vi "SSL Vision Log Player.vi"() -> ()   [LabVIEW 2018]
uses:
  SSL Referee Game Status.ctl
  GUI/IA Robot Line Display.ctl
  Intel/Functions Enum.ctl
  Filters/Estimadores.ctl
  Control/SSL Data Control.ctl
  Control/SSL UDP Address.ctl
  Control/File Player.ctl
  Intel/Command Enum.ctl
  Test/TestModule.ctl
  Util/Select None or Robot.ctl
  DrawTargets.ctl
  Select Personalitys.ctl
  Util/Select Auto None or Robot.ctl
  Intel/AI Parameters.ctl
  grSim/grSim RobotReplacement.ctl
  grSim/grSim_BallReplacement.ctl
  SSL Detection Frame.ctl
  SSL Detection Robot.ctl
  <vilib>/Analysis/Matrix/Datatypes/RealMatrix.ctl
  SSL Detection Ball.ctl
  SSL/SSL Field State.ctl
  <extravilib>/ChannelInstances/Lossy Stream-a[.](u8)/Read With Abort.vi
  <extravilib>/ChannelInstances/Lossy Stream-t'SSL Referee Game Status.ctl'/Write With Abort.vi
  <extravilib>/ChannelInstances/Lossy Stream-bool/Read With Abort.vi
  <extravilib>/ChannelInstances/Lossy Stream-bool/Write With Abort.vi
  <extravilib>/ChannelInstances/Lossy Stream-t'AI Input.ctl'/Write With Abort.vi
  <extravilib>/ChannelInstances/Lossy Stream-c(a[.](t'grSim RobotReplacement.ctl'),t'grSim_BallReplacement.ctl')/Read With Abort.vi
  <extravilib>/ChannelInstances/Lossy Stream-t'AI Input.ctl'/Read With Abort.vi
  <extravilib>/ChannelInstances/Lossy Stream-a[.](bool)/Write With Abort.vi
  <extravilib>/ChannelInstances/Lossy Stream-a[.](i32)/Read With Abort.vi
  <extravilib>/ChannelInstances/Lossy Stream-c(a[.](t'grSim RobotReplacement.ctl'),t'grSim_BallReplacement.ctl')/Write With Abort.vi
  <extravilib>/ChannelInstances/Lossy Stream-a[.](bool)/Read With Abort.vi
  <extravilib>/ChannelInstances/Lossy Stream-a[.](u16)/Read With Abort.vi
  <extravilib>/ChannelInstances/Lossy Stream-a[.](i32)/Write With Abort.vi
  <extravilib>/ChannelInstances/Lossy Stream-t'SSL Field State.ctl'/Read With Abort.vi
  <extravilib>/ChannelInstances/Lossy Stream-t'SSL Referee Game Status.ctl'/Read With Abort.vi
  <extravilib>/ChannelInstances/Lossy Stream-a[.](t'SSL Detection Frame.ctl')/Read With Abort.vi
  <extravilib>/ChannelInstances/Lossy Stream-c(u32,u32,u32,u32,u32,u32,u32,u32,u32,u32,u32,u32,u32,u32)/Read With Abort.vi
  <extravilib>/ChannelInstances/Lossy Stream-t'SSL Field State.ctl'/Write With Abort.vi
  <extravilib>/ChannelInstances/Lossy Stream-a[.](u16)/Write With Abort.vi
  <extravilib>/ChannelInstances/Lossy Stream-a[.](t'SSL Detection Frame.ctl')/Write With Abort.vi
  <extravilib>/ChannelInstances/Lossy Stream-c(u32,u32,u32,u32,u32,u32,u32,u32,u32,u32,u32,u32,u32,u32)/Write With Abort.vi
  <extravilib>/ChannelInstances/Lossy Stream-a[.](u8)/EndpointRead.vi
  <extravilib>/ChannelInstances/Lossy Stream-t'SSL Referee Game Status.ctl'/Endpoint.vi
  <extravilib>/ChannelInstances/Lossy Stream-bool/EndpointRead.vi
  <extravilib>/ChannelInstances/Lossy Stream-bool/Endpoint.vi
  <extravilib>/ChannelInstances/Lossy Stream-t'AI Input.ctl'/Endpoint.vi
  <extravilib>/ChannelInstances/Lossy Stream-c(a[.](t'grSim RobotReplacement.ctl'),t'grSim_BallReplacement.ctl')/EndpointRead.vi
  <extravilib>/ChannelInstances/Lossy Stream-t'AI Input.ctl'/EndpointRead.vi
  <extravilib>/ChannelInstances/Lossy Stream-a[.](bool)/Endpoint.vi
  <extravilib>/ChannelInstances/Lossy Stream-a[.](i32)/EndpointRead.vi
  <extravilib>/ChannelInstances/Lossy Stream-c(a[.](t'grSim RobotReplacement.ctl'),t'grSim_BallReplacement.ctl')/Endpoint.vi
  <extravilib>/ChannelInstances/Lossy Stream-a[.](bool)/EndpointRead.vi
  <extravilib>/ChannelInstances/Lossy Stream-a[.](u16)/EndpointRead.vi
  <extravilib>/ChannelInstances/Lossy Stream-a[.](i32)/Endpoint.vi
  <extravilib>/ChannelInstances/Lossy Stream-t'SSL Field State.ctl'/EndpointRead.vi
  <extravilib>/ChannelInstances/Lossy Stream-t'SSL Referee Game Status.ctl'/EndpointRead.vi
  <extravilib>/ChannelInstances/Lossy Stream-a[.](t'SSL Detection Frame.ctl')/EndpointRead.vi
  <extravilib>/ChannelInstances/Lossy Stream-c(u32,u32,u32,u32,u32,u32,u32,u32,u32,u32,u32,u32,u32,u32)/EndpointRead.vi
  <extravilib>/ChannelInstances/Lossy Stream-t'SSL Field State.ctl'/Endpoint.vi
  <extravilib>/ChannelInstances/Lossy Stream-a[.](u16)/Endpoint.vi
  <extravilib>/ChannelInstances/Lossy Stream-a[.](t'SSL Detection Frame.ctl')/Endpoint.vi
  <extravilib>/ChannelInstances/Lossy Stream-c(u32,u32,u32,u32,u32,u32,u32,u32,u32,u32,u32,u32,u32,u32)/Endpoint.vi
  <extravilib>/ChannelInstances/Lossy Stream-a[.](t'SSL Detection Frame.ctl')/Instantiate.vi
  <extravilib>/ChannelInstances/Lossy Stream-c(u32,u32,u32,u32,u32,u32,u32,u32,u32,u32,u32,u32,u32,u32)/Instantiate.vi
  <extravilib>/ChannelInstances/Lossy Stream-a[.](u8)/Instantiate.vi
  <extravilib>/ChannelInstances/Lossy Stream-a[.](u8)/)Channel.vi
  <resource>/ChannelSupport/_ChannelSupport/WaitIfNeeded.vi
  <extravilib>/ChannelInstances/Lossy Stream-a[.](t'SSL Detection Frame.ctl')/)Channel.vi
  <extravilib>/ChannelInstances/Lossy Stream-c(u32,u32,u32,u32,u32,u32,u32,u32,u32,u32,u32,u32,u32,u32)/)Channel.vi
  <extravilib>/ChannelInstances/Lossy Stream-a[.](i32)/Instantiate.vi
  <extravilib>/ChannelInstances/Lossy Stream-t'SSL Field State.ctl'/Instantiate.vi
  Util/PreviousState.vi
  <extravilib>/ChannelInstances/Lossy Stream-c(a[.](t'grSim RobotReplacement.ctl'),t'grSim_BallReplacement.ctl')/Instantiate.vi
  <extravilib>/ChannelInstances/Lossy Stream-bool/Instantiate.vi
  <extravilib>/ChannelInstances/Lossy Stream-a[.](bool)/Instantiate.vi
  <extravilib>/ChannelInstances/Lossy Stream-t'AI Input.ctl'/Instantiate.vi
  <extravilib>/ChannelInstances/Lossy Stream-bool/)Channel.vi
  <extravilib>/ChannelInstances/Lossy Stream-t'AI Input.ctl'/)Channel.vi
  <extravilib>/ChannelInstances/Lossy Stream-a[.](bool)/)Channel.vi
  <extravilib>/ChannelInstances/Lossy Stream-a[.](i32)/)Channel.vi
  <extravilib>/ChannelInstances/Lossy Stream-c(a[.](t'grSim RobotReplacement.ctl'),t'grSim_BallReplacement.ctl')/)Channel.vi
  <extravilib>/ChannelInstances/Lossy Stream-a[.](u16)/Instantiate.vi
  <extravilib>/ChannelInstances/Lossy Stream-t'SSL Field State.ctl'/)Channel.vi
  <extravilib>/ChannelInstances/Lossy Stream-a[.](u16)/)Channel.vi
  <extravilib>/ChannelInstances/Lossy Stream-t'SSL Referee Game Status.ctl'/Instantiate.vi
  <extravilib>/ChannelInstances/Lossy Stream-t'SSL Referee Game Status.ctl'/)Channel.vi
  <extravilib>/ChannelInstances/Lossy Stream-t'SSL Referee Game Status.ctl'.lvlib
  <extravilib>/ChannelInstances/Lossy Stream-t'AI Input.ctl'.lvlib
  <extravilib>/ChannelInstances/Lossy Stream-a[.](u8).lvlib
  <vilib>/Analysis/Matrix/NI_Matrix.lvlib
  <extravilib>/ChannelInstances/Lossy Stream-a[.](i32).lvlib
  <extravilib>/ChannelInstances/Lossy Stream-t'SSL Field State.ctl'.lvlib
  <extravilib>/ChannelInstances/Lossy Stream-bool.lvlib
  <extravilib>/ChannelInstances/Lossy Stream-a[.](u16).lvlib
  <extravilib>/ChannelInstances/Lossy Stream-c(a[.](t'grSim RobotReplacement.ctl'),t'grSim_BallReplacement.ctl').lvlib
  <extravilib>/ChannelInstances/Lossy Stream-a[.](bool).lvlib
  <extravilib>/ChannelInstances/Lossy Stream-c(u32,u32,u32,u32,u32,u32,u32,u32,u32,u32,u32,u32,u32,u32).lvlib
  <extravilib>/ChannelInstances/Lossy Stream-a[.](t'SSL Detection Frame.ctl').lvlib
panel:
  in  "Robô":i32
  in  "Liga/Desliga":bool
  out "Camera Decode FPS":dbl
  out "Filter Observation FPS":dbl
  out "2D Picture":picture
  out "Direct\nkick":bool
  out "Intel FPS":dbl
  in  "CamerasToIgnore":dbl[](array[numeric])=[-1.0, -1.0, -1.0, -1.0]
  in  "Test tab control":enum32{"Modo Teste", "GrSim Modo Teste"}(tab)
  in  "test module":T1={"Goto"="None", "ZigZag 0"=["None", "None", "None", "None", "None", "None", "None", "None", "None"], "Kicker"="None", "Vel_kick"=100.0, "Kick"=FALSE, "Modo Teste?"=FALSE, "GoTo point"=[], "zigzag points"=[{"x"=300.0, "y"=2000.0}, {"x"=300.0, "y"=-2000.0}], " id vel"=1, "Dribble"=FALSE, "Gravando"=FALSE, "output xy"=4.0, "output\nangle"=4.0, "angle\nzigzag"=32.5, "output inc"=2.0, "Accel"=6.0, "DesAccel"=1.35}
  in  "Test Mode On":bool
  in  "Generate new random points":bool
  in  "Number of Points":i32=100
  in  "Replace Robots":bool=TRUE
  in  "reset":bool
  out "Completed Generation":bool
  in  "id":i32=5
  out "kick num":i32
  in  "Test Attacker":bool
  in  "Modulo Velocidade":dbl=2000.0 format="%#_13g"
  in  "Test Passe":bool
  in  "Debug":bool
  in  "GoTo Navigation":bool
  in  "Pinned":T3={"Attc"="Auto", "Strk"="Auto", "Def"=["Auto", "Auto", "Auto"]}
  in  "Draw Targets?":T5={"Attacker"=TRUE, "Striker"=TRUE, "Goalie"=TRUE, "Defender"=TRUE, "kick"=TRUE, "Est Ball"=TRUE, "Est Robot"=FALSE, "Path S"=FALSE, "Path C"=FALSE, "Dngr.Enemy"=TRUE}
  in  "SSL Data":T6={"Modo"=TRUE, "SSL UDP RX"={"Port:"=10006, "Server IP:"="224.5.23.2", "Local IP:"="10.4.0.248", "RX"=TRUE}, "RefBox UDP RX"={"Port:"=10003, "Server IP:"="224.5.23.1", "Local IP:"="10.4.0.248", "RX"=TRUE}, "Reprodução de Arquivo"={"file path (use dialog)"=path "E:/Media/2016-07-01_cmdragons_immortals.log", "size (in bytes)"=0, "offset (in bytes)"=0, "Slide"=0.0, "Play"=FALSE, "Time Stamp"=timestamp(0 s since 1904-01-01), "Playing"=FALSE}} {"Reprodução de Arquivo"."Time Stamp" format="%<%.3X %x>T"; "Reprodução de Arquivo"."Slide" min=0 max=1 scale=0.0..1.0; "Reprodução de Arquivo"."offset (in bytes)" format="%.3p"; "Reprodução de Arquivo"."size (in bytes)" format="%.3p"}
  out "error out 5":errorcluster
  out "error out 3":errorcluster
  out "Pass":bool
  out "IA command":T9
  in  "ignora esquerda?":bool
  in  "ignora lado?":bool
  in  "atacando ao contrário?":bool
  in  "Defense stretch":i32=2000
  in  "Defense width":i32=1000
  in  "Estimador":T10=enum."Kalman"
  out "Role Playing \nFPS":dbl
  out "Total Delay":dbl format="%#.5g"
  in  "Goalie":string(combo)="0"
  in  "Command":string(combo)="Auto"
  in  "Time":enum16{"Azul", "Amarelo"}(ring) caption="Enum"
  in  "Lado":enum16{"Esquerdo", "Direito"}(ring) caption="Enum"
  in  "Role Decisor":enum16{"Simple Role Decisor", "No Role Decisor"}(ring)
  out "bot velocity":dbl(graph)
  out "ball":dbl(graph)
  in  "Tab Control":enum32{"RX Info", "TX info", "AI Parameters"}(tab)=enum."AI Parameters"
  out "GUI Robot Array":T11[](array[typedef])
  out "Game Status":T13={"Stage"="Normal First Half Pre", "Command"="Stop", "Time Left"=0.0, "Yellow Team"="", "Blue Team"="", "Yellow Score"=0, "Blue Score"=0, "Yellow Red Cards"=0, "Blue Red Cards"=0, "Yellow Yellow Cards"=0, "Blue Yellow Cards"=0, "Yellow Timeouts Left"=0, "Blue Timeouts Left"=0, "Yellow Timeout Remaining"=0.0, "Blue Timeout Remaining"=0.0, "Yellow Goalie Id"=0, "Blue Goalie Id"=0, "Time"=timestamp(2082758400 s since 1904-01-01)} {"Time" format="%<%.3X %x>T"; "Blue Timeout Remaining" format="%<%M:%S>t"; "Yellow Timeout Remaining" format="%<%M:%S>t"; "Time Left" format="%<%M:%S>t"}
  in  "Serial TX":bool
  in  "UDP GrSim TX":bool=TRUE
  in  "Address:":string="127.0.0.1"
  in  "Port:":u16=20011
  in  "Porta:":refnum<visa-resource-name>
  out "Comm TX FPS":dbl
  in  "UDP SOS TX":bool
  in  "SOS Address:":string="192.168.0.101"
  in  "SOS Port:":u16=10021
  in  "SOS Port: 2":u16=10025
  out "grSim replacement":cluster{"robots":T14[], "ball":T15}
  out "replace active":bool
  in  "AI Parameters":T16={"GotoKick"={"Dist do cone a frente"=0.0, "attacker farback"=1300.0, "Perto"=300.0, "min dist to kick"=140.0, "kick eps"=0.15, "Time to transition"=0.3}, "Attacker"={"CC chute"=0.7, "CC passe"=0.65, "Kick Force"=85.0, "ball-robot Kick"=300.0, "ball-robot Pass"=350.0, "drible\nAttk"=FALSE}, "Defender"={"D max"=1500.0, "Vel p/ robô av"=0.2, "Kick Force"=100.0, "D atk-def"=400.0, "D farback"=300.0, "drible\ndef"=FALSE, "drible\ngoalie"=FALSE}, "Timeout"={"Field/v in x"=6.0, "Dist Robots"=300, "Dist up in y"=300}, "Pose Striker"={"dist"=650.0, "Numeric"=-4.0, "dist 2"=650.0, "drible\nstriker"=TRUE}, "Dist Stop"=700.0, "D ball out"=200, "D central gap "=125.0, "T pass"=5.0, "Force ++"=5.0, "range kick"=60.0, "Chute alto"=TRUE, "Marcador novo"=TRUE, "drible"=FALSE, "D drible"=500.0} {"D drible" format="%#_13g"; "D central gap" format="%#_13g"; "Dist Stop" format="%#_13g"; "Pose Striker"."Numeric" format="%#_13g"; "Defender"."Kick Force" format="%#_13g"; "Defender"."Vel p/ robô av" format="%#_13g"; "Attacker"."ball-robot Kick" format="%#_13g"; "Attacker"."Kick Force" format="%#_13g"; "Attacker"."CC passe" format="%#_13g"; "Attacker"."CC chute" format="%#_13g"; "GotoKick"."min dist to kick" format="%#_13g"; "GotoKick"."Perto" format="%#_13g"; "GotoKick"."attacker farback" format="%#_13g"; "GotoKick"."Dist do cone a frente" format="%#_13g"}
  in  "D posse":dbl=220.0
  in  "Tol ang posse":dbl=0.3
  in  "D toque":dbl=130.0
  in  "Qtd Min p/ Stk":dbl=4.0
  in  "Mais perigoso/segundo\nmais perigoso":T17(ring)
  in  "Defesa nova/antiga":T18(ring)
  in  "D bola anda":dbl=2.0
  # "Ligue o Test Mode\nprimeiro"
  # "UDP"
  # "LOG"
  # "Score"
  # "Red Cards"
  # "Yellow Cards"
  # "Timeouts Left"
  # "Timeout Remaining"
  # "Goalie ID"
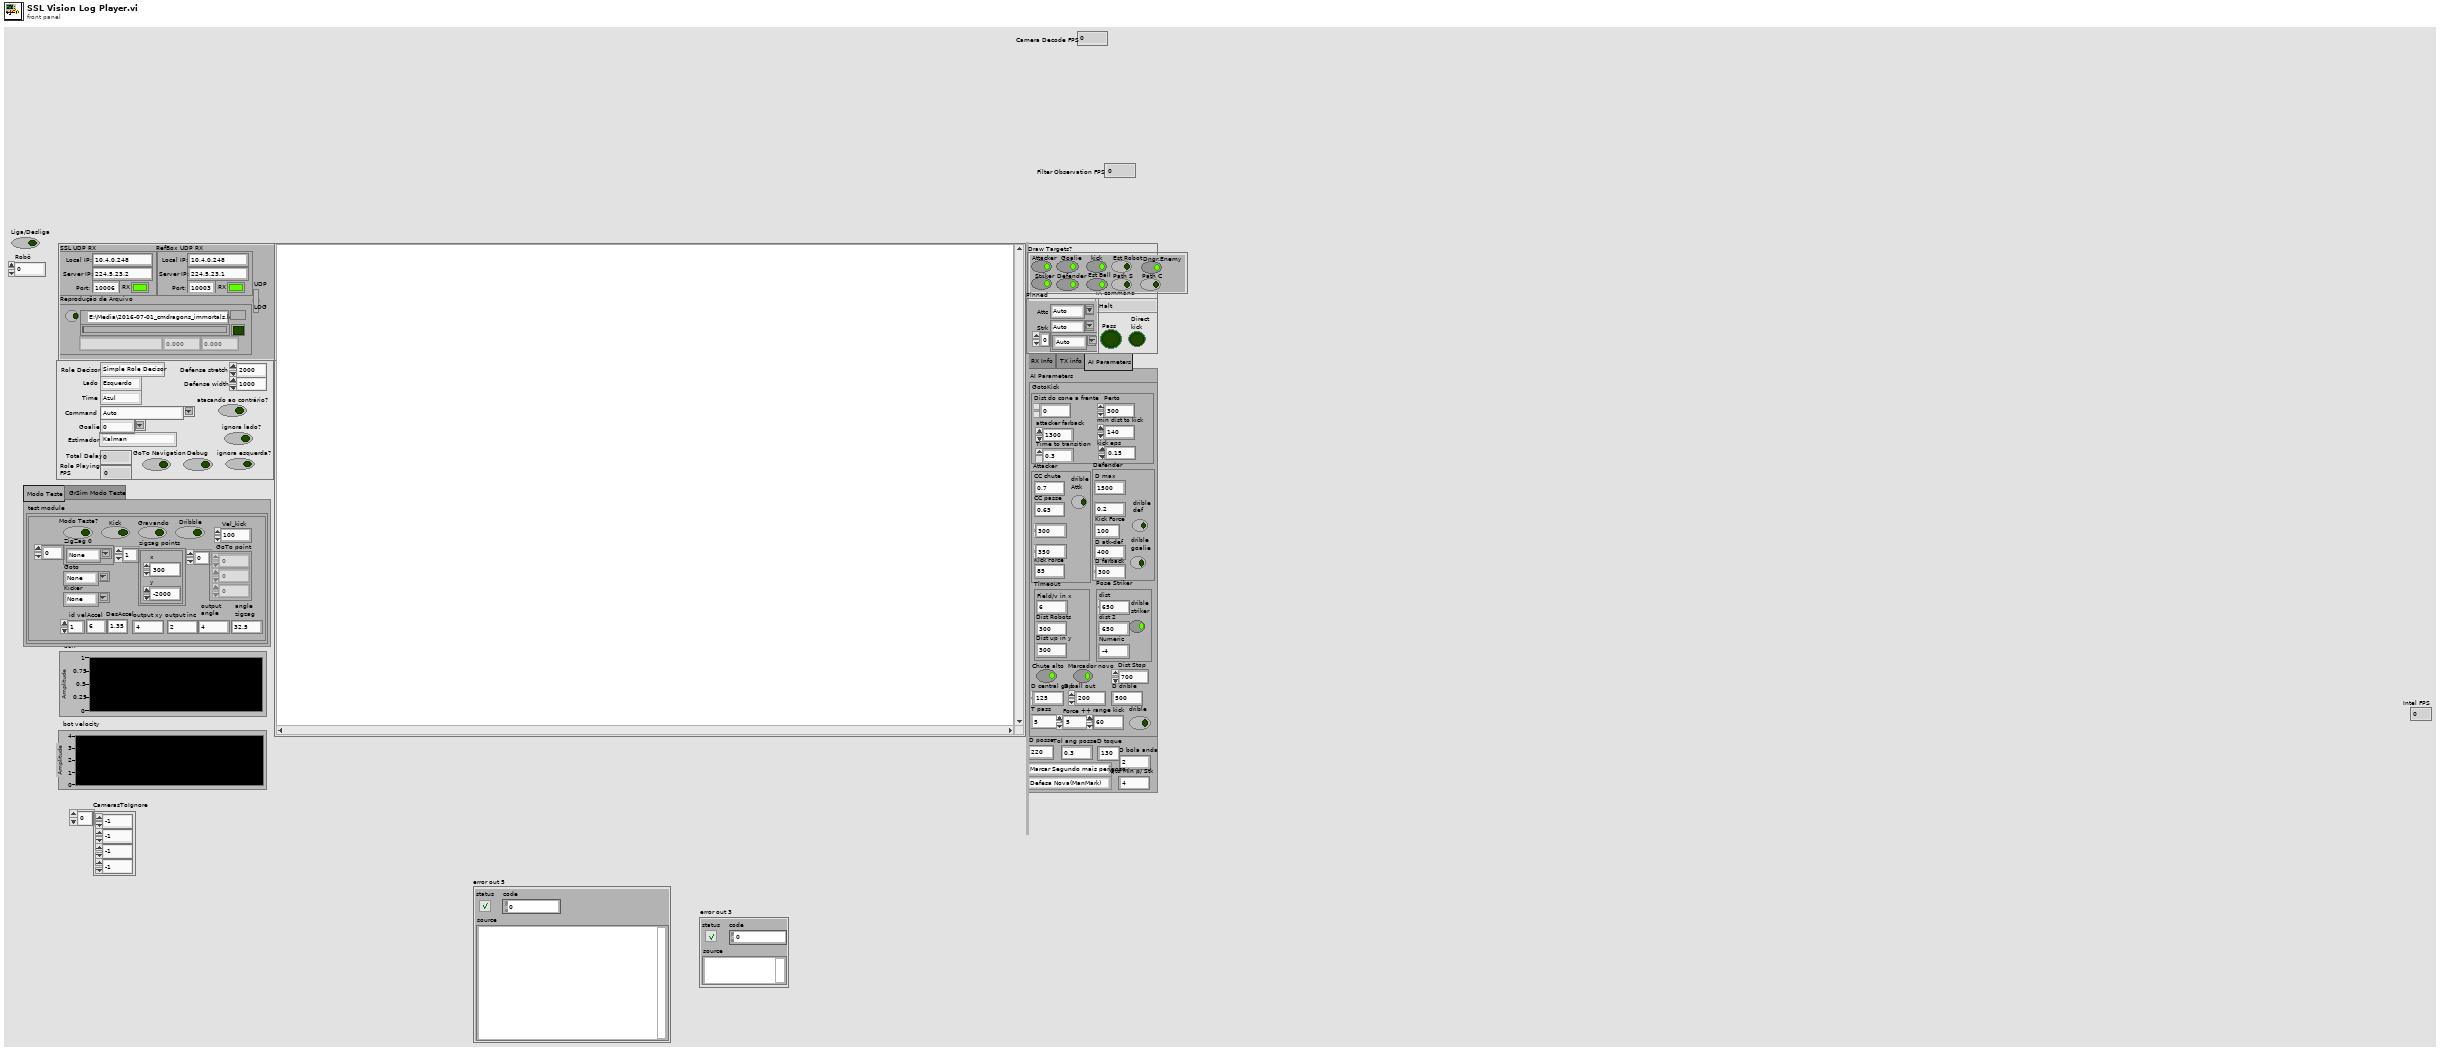
[diagram p1: front panel]
types:
  T1 = typedef "TestModule.ctl" = cluster{"Goto":T2, "ZigZag 0":T2[], "Kicker":T2, "Vel_kick":dbl, "Kick":bool, "Modo Teste?":bool, "GoTo point":dbl[], "zigzag points":cluster{"x":dbl, "y":dbl}[], " id vel":u32, "Dribble":bool, "Gravando":bool, "output xy":dbl, "output\nangle":dbl, "angle\nzigzag":dbl, "output inc":dbl, "Accel":dbl, "DesAccel":dbl}
  T2 = typedef "Select None or Robot.ctl" = string
  T3 = typedef "Select Personalitys.ctl" = cluster{"Attc":T4, "Strk":T4, "Def":T4[]}
  T4 = typedef "Select Auto None or Robot.ctl" = string
  T5 = typedef "DrawTargets.ctl" = cluster{"Attacker":bool, "Striker":bool, "Goalie":bool, "Defender":bool, "kick":bool, "Est Ball":bool, "Est Robot":bool, "Path S":bool, "Path C":bool, "Dngr.Enemy":bool}
  T6 = typedef "SSL Data Control.ctl" = cluster{"Modo":bool, "SSL UDP RX":T7, "RefBox UDP RX":T7, "Reprodução de Arquivo":T8}
  T7 = typedef "SSL UDP Address.ctl" = cluster{"Port:":u16, "Server IP:":string, "Local IP:":string, "RX":bool}
  T8 = typedef "File Player.ctl" = cluster{"file path (use dialog)":path, "size (in bytes)":i64, "offset (in bytes)":i64, "Slide":sgl, "Play":bool, "Time Stamp":timestamp, "Playing":bool}
  T9 = typedef "Command Enum.ctl" = enum16{"Halt", "Stop", "Force Start", "PKA Normal Start", "Prepare Kickoff Ally", "PKE Normal Start", "Prepare Kickoff Enemy", "Prepare Penalty Ally", "PPA Normal Start", "Prepare Penalty Enemy", "PPE Normal Start", "Direct Free Enemy", "Direct Free Ally", "Indirect Free Enemy", "Indirect Free Ally", "Timeout Enemy", "Timeout Ally", "Goal Enemy", "Goal Ally", "Ball Placement Enemy", "Ball Placement Ally", "Normal Half Time", "Extra Time Break", "Extra Half Time", "None", "Post Game"}
  T10 = typedef "Estimadores.ctl" = enum16{"Nenhum", "Simples", "Kalman"}
  T11 = typedef "IA Robot Line Display.ctl" = cluster{"ID":dbl, "function":T12, "dribble":bool}
  T12 = typedef "Functions Enum.ctl" = enum16{"Attacker", "Goalie", "Defender", "Striker", "Goto 0", "Dummy", "Kicker", "ZigZag 0", "ZigZag 1", "ZigZag 2", "ZigZag 3", "ZigZag 4", "ZigZag 5", "ZigZag 6", "ZigZag 7", "ZigZag 8", ""}
  T13 = typedef "SSL Referee Game Status.ctl" = cluster{"Stage":string, "Command":string, "Time Left":dbl, "Yellow Team":string, "Blue Team":string, "Yellow Score":u32, "Blue Score":u32, "Yellow Red Cards":u32, "Blue Red Cards":u32, "Yellow Yellow Cards":u32, "Blue Yellow Cards":u32, "Yellow Timeouts Left":u32, "Blue Timeouts Left":u32, "Yellow Timeout Remaining":dbl, "Blue Timeout Remaining":dbl, "Yellow Goalie Id":u32, "Blue Goalie Id":u32, "Time":timestamp}
  T14 = typedef "grSim RobotReplacement.ctl" = cluster{"x":dbl, "y":dbl, "dir":dbl, "yellowteam":bool, "id":u32}
  T15 = typedef "grSim_BallReplacement.ctl" = cluster{"x":dbl, "y":dbl, "vx":dbl, "vy":dbl}
  T16 = typedef "AI Parameters.ctl" = cluster{"GotoKick":cluster{"Dist do cone a frente":dbl, "attacker farback":dbl, "Perto":dbl, "min dist to kick":dbl, "kick eps":dbl, "Time to transition":dbl}, "Attacker":cluster{"CC chute":dbl, "CC passe":dbl, "Kick Force":dbl, "ball-robot Kick":dbl, "ball-robot Pass":dbl, "drible\nAttk":bool}, "Defender":cluster{"D max":dbl, "Vel p/ robô av":dbl, "Kick Force":dbl, "D atk-def":dbl, "D farback":dbl, "drible\ndef":bool, "drible\ngoalie":bool}, "Timeout":cluster{"Field/v in x":dbl, "Dist Robots":u32, "Dist up in y":u32}, "Pose Striker":cluster{"dist":dbl, "Numeric":dbl, "dist 2":dbl, "drible\nstriker":bool}, "Dist Stop":dbl, "D ball out":i32, "D central gap ":dbl, "T pass":dbl, "Force ++":dbl, "range kick":dbl, "Chute alto":bool, "Marcador novo":bool, "drible":bool, "D drible":dbl}
  T17 = enum16{"Marcar Segundo mais perigoso", "Marcar o mais perigoso"}
  T18 = enum16{"Defesa Nova(ManMark)", "Defesa Antiga(Barreira)"}
  T19 = typedef "Lossy Stream-a[.](u8).lvlib/)Channel.ctl" = refnum<queue>
  T20 = typedef "SSL Referee.ctl" = cluster{"packet_\ntimestamp":u64, "stage":u64, "stage_time_left":i32, "command ":u64, "command_\ncounter ":u32, "command_\ntimestamp":u64, "yellow team info":T21, "blue team info":T21, "Point":cluster{"x":sgl, "y":sgl}}
  T21 = typedef "SSL Referee Team Info.ctl" = cluster{"name":string, "score":u32, "red_cards":u32, "yellow_cards_time":u32[], "yellow_cards":u32, "timeout":u32, "timeout_times":u32, "goalie":u32}
  T22 = typedef "Lossy Stream-t'SSL Referee Game Status.ctl'.lvlib/)Channel.ctl" = refnum<queue>
  T23 = typedef "SSL Detection Frame.ctl" = cluster{"frame_number":u32, "t_capture":dbl, "t_sent":dbl, "camera_id":u32, "robots_yellow":T24[], "robots_blue":T24[], "balls":T26[], "Valid":bool, "Time Stamp":timestamp}
  T24 = typedef "SSL Detection Robot.ctl" = cluster{"x":sgl, "robot_id":u32, "confidence":sgl, "y":sgl, "orientation":sgl, "pixel_x":sgl, "pixel_y":sgl, "height":sgl, "Valid":bool, "Time Stamp":timestamp, "x_k|k":T25, "Pk|k":T25, "Previous Time Stamp":timestamp, "R":T25}
  T25 = typedef "NI_Matrix.lvlib/RealMatrix.ctl" = dbl[][]
  T26 = typedef "SSL Detection Ball.ctl" = cluster{"x":sgl, "area":u32, "confidence":sgl, "y":sgl, "z":sgl, "pixel_x":sgl, "pixel_y":sgl, "Valid":bool, "Time Stamp":timestamp, "x_k|k":T25, "Pk|k":T25, "Id":u32, "Previous Time Stamp":timestamp, "R":T25}
  T27 = cluster{"line_width":u32, "field_length":u32, "field_width":u32, "boundary_width":u32, "referee_width":u32, "goal_width":u32, "goal_depth":u32, "goal_wall_width":u32, "center_circle_radius":u32, "defense_radius":u32, "defense_stretch":u32, "free_kick_from_defense_dist":u32, "penalty_spot_from_field_line_dist":u32, "penalty_line_from_spot_dist":u32}
  T28 = typedef "Lossy Stream-c(u32,u32,u32,u32,u32,u32,u32,u32,u32,u32,u32,u32,u32,u32).lvlib/)Channel.ctl" = refnum<queue>
  T29 = typedef "Lossy Stream-a[.](t'SSL Detection Frame.ctl').lvlib/)Channel.ctl" = refnum<queue>
  T30 = typedef "SSL Field State.ctl" = cluster{"Detection Frame Out":T23, "Field Size Out":cluster{"line_width":u32, "field_length":u32, "field_width":u32, "boundary_width":u32, "referee_width":u32, "goal_width":u32, "goal_depth":u32, "goal_wall_width":u32, "center_circle_radius":u32, "defense_radius":u32, "defense_stretch":u32, "free_kick_from_defense_dist":u32, "penalty_spot_from_field_line_dist":u32, "penalty_line_from_spot_dist":u32}, "Received Time Stamp":timestamp}
  T31 = typedef "AI Input.ctl" = cluster{"our_robots":T32[], "enemy_robots":T32[], "balls":T36[], "geometry":T37, "IA Judge":T38, "Received Timestamp":timestamp, "Events":T39}
  T32 = typedef "AI Robot.ctl" = cluster{"id":u32, "function":T12, "x":dbl, "y":dbl, "orientation":dbl, "v_tangent":dbl, "v_normal":dbl, "v_ang":dbl, "kick_x":dbl, "kick_z":dbl, "dribble":bool, "Timestamp":timestamp, "estimatives":cluster{"est_v_tangent":dbl, "est_v_normal":dbl, "est_vx":dbl, "est_vy":dbl, "Pos Robot Est":dbl[]}, "dest_x_kick":dbl, "dest_y_kick":dbl, "Gap Coord":dbl[], "States":T33, "Path ":dbl[][], "Path  Smooth":dbl[][], "Dest":T34}
  T33 = typedef "AttackerStates.ctl" = enum16{"Pass", "GoToTangent", "BallGetting", "GoToKick", ""}
  T34 = typedef "PathDests.ctl" = T35[]
  T35 = typedef "PathDest.ctl" = cluster{"dest_x":dbl, "dest_y":dbl, "dest_orientation":dbl, "dest_vel":dbl}
  T36 = typedef "AI Ball.ctl" = cluster{"x":dbl, "y":dbl, "timestamp":timestamp, "Vel_x":dbl, "Vel_y":dbl, "Pos Bola Est":dbl[]}
  T37 = typedef "Field Size.ctl" = cluster{"line_width":u32, "field_length":u32, "field_width":u32, "boundary_width":u32, "referee_width":u32, "goal_width":u32, "goal_depth":u32, "goal_wall_width":u32, "center_circle_radius":u32, "defense_radius":u32, "defense_stretch":u32, "free_kick_from_defense_dist":u32, "penalty_spot_from_field_line_dist":u32, "penalty_line_from_spot_dist":u32}
  T38 = typedef "AI Judge.ctl" = cluster{"stage":string, "command":string, "our_goalie_id":dbl, "enemy_goalie_id":dbl, "command enum":T9, "Time":enum16{"Azul", "Amarelo"}}
  T39 = typedef "Events.ctl" = cluster{"Touch":bool, "Ball out":bool, "id touch":dbl, "Ball out of \nVision":bool, "Ball inside \nGoalie area":bool, "Robot not responding":bool, "Robots responding status":dbl[], "Enemy Ball \nPossession":bool, "Pass State":bool, "id end of pass":dbl, "Kick":bool, "Id ini Possession":dbl, "Ball Possesion":bool, "Id Possesion":dbl, "Direct Kick":bool}
  T40 = typedef "Lossy Stream-a[.](u16).lvlib/)Channel.ctl" = refnum<queue>
  T41 = typedef "Lossy Stream-t'SSL Field State.ctl'.lvlib/)Channel.ctl" = refnum<queue>
  T42 = typedef "Lossy Stream-a[.](i32).lvlib/)Channel.ctl" = refnum<queue>
  T43 = typedef "Lossy Stream-t'AI Input.ctl'.lvlib/)Channel.ctl" = refnum<queue>
  T44 = typedef "Lossy Stream-bool.lvlib/)Channel.ctl" = refnum<queue>
  T45 = typedef "Lossy Stream-a[.](bool).lvlib/)Channel.ctl" = refnum<queue>
  T46 = typedef "Lossy Stream-c(a[.](t'grSim RobotReplacement.ctl'),t'grSim_BallReplacement.ctl').lvlib/)Channel.ctl" = refnum<queue>
  T47 = typedef "grSim Robot Command.ctl" = cluster{"id":u32, "kickspeedx":sgl, "kickspeedz":sgl, "veltangent":sgl, "velnormal":sgl, "velangular":sgl, "spinner":bool, "wheelspeed":bool, "wheel1":sgl, "wheel2":sgl, "wheel3":sgl, "wheel4":sgl}
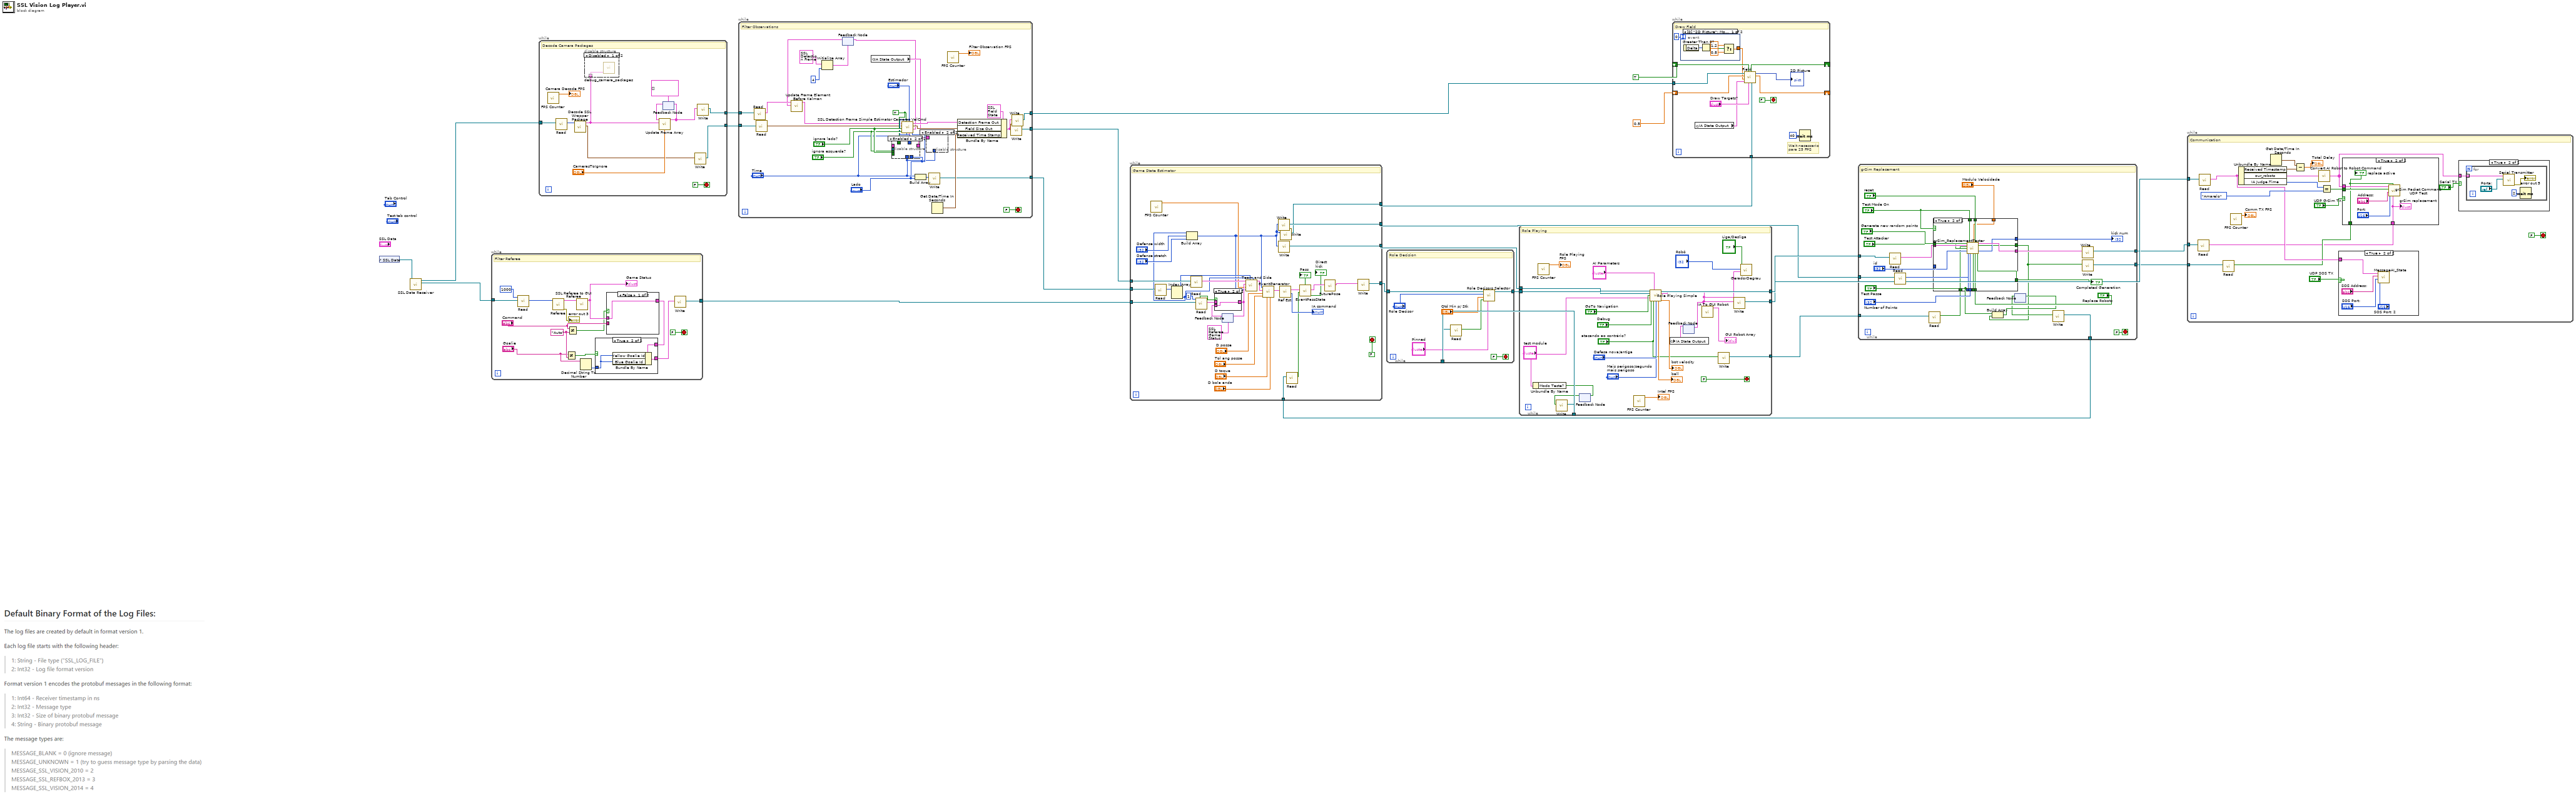
[diagram p0: block diagram]
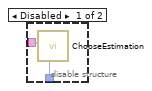
[diagram p3: hidden frame]
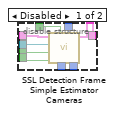
[diagram p4: hidden frame]
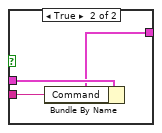
[diagram p6: hidden frame]
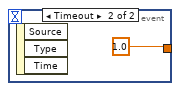
[diagram p7: hidden frame]
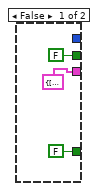
[diagram p9: hidden frame]
diagram:
  n1 = control-ref of="SSL Data"() -> (w18:refnum<vi>)
  n2 = call "SSL Data Receiver.vi"("SSL Data 2"=w18) -> ("SSL RefBox"=w19:T19, "SSL Vision"=w3:T19)  [unwired: 9 in]
  n3 = while {
    tunnel: w19 -> [w26]
    tunnel: [w36] -> w21
    stop <- FALSE stop-if-true
    w32 = "Auto" ("y")
    # "Filter Referee"
    n4 = call <extravilib>:"Read.vi"("channel"=w26, "timeout in ms (-1)"=1000) -> ("element"=w25:u8[])  [unwired: 4 in, 5 out]
    n5 = call "Referee.vi"("element"=w25) -> ("output cluster"=w37:T20, "error out"=→"error out 3":errorcluster)  [unwired: 13 in]
    n6 = Not Equal?(x="Goalie", y=w32) -> (x != y?=w31:bool)
    n7 = Not Equal?(x="Command", y=w32) -> (x != y?=w33:bool)
    n8 = call "SSL Referee to GUI Referee.vi"("SSL Game Status"=w37) -> ("GUI Game Status"=w35:T13)  [unwired: 10 in]
    "Game Status" <- w35
    n9 = Decimal String To Number(string="Goalie") -> (number=w27:i32)  [unwired: 2 in, 1 out]
    n10 = case shown="False" w33 {
      tunnel: w35 -> [w44 w47]
      tunnel: [w44 w46] -> w30
      tunnel: "Command" -> [_ w45]
      frame False {
      }
      frame True {
        n11 = Bundle By Name(cluster=w47, "Command"=w45) -> (w46:T13)
      }
    }
    n12 = case shown="True" w31 {
      tunnel: w30 -> [w40 w43]
      tunnel: [w40 w42] -> w29
      tunnel: w27 -> [_ w41]
      frame False {
      }
      frame True {
        n13 = Bundle By Name(cluster=w43, "Yellow Goalie Id"=w41, "Blue Goalie Id"=w41) -> (w42:T13)
      }
    }
    n14 = call <extravilib>:"Write.vi"("element"=w29) -> ("channel"=w36:T22)  [unwired: 8 in, 2 out]
  }
  n15 = while {
    tunnel: w3 -> [w58]
    tunnel: [w54] -> w2
    tunnel: [w53] -> w1
    stop <- FALSE stop-if-true
    # "Decode Camera Packages"
    n16 = call "FPS Counter.vi"() -> ("Numeric"=→"Camera Decode FPS":dbl)  [unwired: 11 in]
    n17 = call <extravilib>:"Read.vi"("channel"=w58) -> ("element"=w59:u8[])  [unwired: 5 in, 5 out]
    n18 = call "Decode SSL Wrapper Package.vi"("unsigned byte array"=w59) -> ("Field Size"=w55:T27, "Detection Frame"=w49:T23)  [unwired: 7 in, 2 out]
    n19 = disable-structure shown="Disabled" {
      disable-tunnel: w49 -> [w60 _]
      frame Disabled {
        n20 = call "debug_camera_packages.vi"("Detection Frame"=w60) -> ()  [unwired: 11 in]
      }
      frame Enabled {
      }
    }
    n21 = feedback #1(T23[] [] ("element")) -> (w51:T23[])
    n22 = call "Update Frame Array.vi"("CamerasToIgnore"="CamerasToIgnore", "Detection Frame In"=w49, "Array Detection Frame In"=w51) -> ("Detection Frame In out"=w48:T23[])  [unwired: 8 in]
    n23 = feedback-in #1(w48) -> ()
    n24 = call <extravilib>:"Write.vi"("element"=w55) -> ("channel"=w54:T28)  [unwired: 8 in, 2 out]
    n25 = call <extravilib>:"Write.vi"("element"=w48) -> ("channel"=w53:T29)  [unwired: 8 in, 2 out]
  }
  n26 = while {
    tunnel: [w85] -> w14
    tunnel: [w84] -> w13
    tunnel: [w73] -> w5
    tunnel: w2 -> [w71]
    tunnel: w1 -> [w69]
    stop <- FALSE stop-if-true
    w79 = TRUE ("Enable")
    # "Filter Observations"
    n27 = call <extravilib>:"Read.vi"("channel"=w69) -> ("element"=w66:T23[])  [unwired: 5 in, 5 out]
    n28 = call <extravilib>:"Read.vi"("channel"=w71) -> ("element"=w70:T27)  [unwired: 5 in, 5 out]
    n29 = Initialize Array(T23 {"frame_number"=0, "t_capture"=0.0, "t_sent"=0.0, "camera_id"=0, "robots_yellow"=[], "robots_blue"=[], "balls"=[], "Valid"=FALSE, "Time Stamp"=timestamp(0 s since 1904-01-01)} ("Detection Frame"), 4 ("dimension size")) -> (w61:T23[])
    n30 = feedback #2(w61) -> (w64:T23[])
    n31 = call "Update Frame Element Before Kalman.vi"("Old Array With Kalman"=w64, "New Array"=w66) -> ("Detection Frame In out"=w65:T23[])  [unwired: 9 in]
    n32 = global read "PreviousState.vi" "IA State Output"() -> (w68:T31)
    n33 = disable-structure shown="Enabled" {
      disable-tunnel: _ -> [w100 _]
      disable-tunnel: _ -> [w99 _]
      disable-tunnel: "ignora lado?" -> [w98 _]
      disable-tunnel: "ignora esquerda?" -> [w97 _]
      disable-tunnel: "Estimador" -> [w96 _]
      disable-tunnel: w79 -> [w95 _]
      disable-tunnel: [w94 _] -> w78
      disable-tunnel: "Lado" -> [w93 _]
      disable-tunnel: "Time" -> [w92 _]
      frame Disabled {
        n34 = call "SSL Detection Frame Simple Estimator Cameras.vi"("Lado"=w93, "Estimador"=w96, "Time"=w92, "Enable"=w95, "ignora esquerda?"=w97, "ignora lado?"=w98, "Field Size"=w99, "Detection Frame In"=w100) -> ("Detection Frame Out"=w94:T23)  [unwired: 2 in, 1 out]
      }
      frame Enabled {
      }
    }
    n35 = call "SSL Detection Frame Simple Estimator Cameras VelCmd.vi"("Lado"="Lado", "IA State Input"=w68, "Estimador"="Estimador", "Time"="Time", "Enable"=w79, "ignora esquerda?"="ignora esquerda?", "ignora lado?"="ignora lado?", "Field Size"=w70, "Detection Frame In"=w65) -> ("Frame Array"=w67:T23[], "Field Size Out"=w86:T27, "Detection Frame Out"=w75:T23)
    n36 = feedback-in #2(w67) -> ()
    n37 = Build Array("Time", "Lado") -> (w83:u16[])
    n38 = disable-structure shown="Enabled" {
      disable-tunnel: w78 -> [w91 _]
      disable-tunnel: "Time" -> [w90 _]
      frame Disabled {
        n39 = call "ChooseEstimation.vi"("Time"=w90, "Detection Frame Kalman"=w91) -> ()  [unwired: 9 in, 1 out]
      }
      frame Enabled {
      }
    }
    n40 = call <extravilib>:"Write.vi"("element"=w83) -> ("channel"=w84:T40)  [unwired: 8 in, 2 out]
    n41 = Get Date/Time In Seconds() -> (seconds since 1Jan1904=w87:timestamp)
    n42 = call "FPS Counter.vi"() -> ("Numeric"=→"Filter Observation FPS":dbl)  [unwired: 11 in]
    n43 = Bundle By Name(cluster=T30 {"Detection Frame Out"={"frame_number"=0, "t_capture"=0.0, "t_sent"=0.0, "camera_id"=0, "robots_yellow"=[], "robots_blue"=[], "balls"=[], "Valid"=FALSE, "Time Stamp"=timestamp(0 s since 1904-01-01)}, "Field Size Out"={"line_width"=0, "field_length"=0, "field_width"=0, "boundary_width"=0, "referee_width"=0, "goal_width"=0, "goal_depth"=0, "goal_wall_width"=0, "center_circle_radius"=0, "defense_radius"=0, "defense_stretch"=0, "free_kick_from_defense_dist"=0, "penalty_spot_from_field_line_dist"=0, "penalty_line_from_spot_dist"=0}, "Received Time Stamp"=timestamp(0 s since 1904-01-01)}, "Detection Frame Out"=w75, "Field Size Out"=w86, "Received Time Stamp"=w87) -> (w74:T30)
    n44 = call <extravilib>:"Write.vi"("element"=w74) -> ("channel"=w85:T41)  [unwired: 8 in, 2 out]
    n45 = call <extravilib>:"Write.vi"("element"=w74) -> ("channel"=w73:T41)  [unwired: 8 in, 2 out]
  }
  n46 = while {
    tunnel: w21 -> [w135]
    tunnel: [w129] -> w17
    tunnel: [w122] -> w15
    tunnel: w14 -> [w114]
    tunnel: w13 -> [w112]
    tunnel: w10 -> [w105]
    tunnel: [w103] -> w6
    tunnel: [w101] -> w4
    stop <- FALSE stop-if-true
    # "Game State Estimator"
    n47 = call "FPS Counter.vi"() -> ("Numeric"=w107:dbl)  [unwired: 11 in]
    n48 = call <extravilib>:"Read.vi"("channel"=w112) -> ("element"=w111:u16[])  [unwired: 5 in, 5 out]
    n49 = Index Array(array=w111) -> (element #1=w110:u16, element #2=w109:u16)  [unwired: 2 in]
    n50 = Build Array(w109, "Defense width", "Defense stretch") -> (w102:i32[])
    n51 = call <extravilib>:"Read.vi"("channel"=w114) -> ("element"=w113:T30)  [unwired: 5 in, 5 out]
    n52 = call <extravilib>:"Read.vi"("channel"=w135, "timeout in ms (-1)"=1) -> ("element"=w132:T13, "timed out?"=w133:bool)  [unwired: 4 in, 4 out]
    n53 = feedback #3(T13 {"Stage"="First Half", "Command"="Stop", "Time Left"=0.0, "Yellow Team"="", "Blue Team"="", "Yellow Score"=0, "Blue Score"=0, "Yellow Red Cards"=0, "Blue Red Cards"=0, "Yellow Yellow Cards"=0, "Blue Yellow Cards"=0, "Yellow Timeouts Left"=0, "Blue Timeouts Left"=0, "Yellow Timeout Remaining"=0.0, "Blue Timeout Remaining"=0.0, "Yellow Goalie Id"=0, "Blue Goalie Id"=0, "Time"=timestamp(0 s since 1904-01-01)} ("element")) -> (w131:T13)
    n54 = case shown="True" w133 {
      tunnel: w132 -> [w137 _]
      tunnel: [w137 w138] -> w130
      tunnel: w131 -> [_ w138]
      frame False {
      }
      frame True {
      }
    }
    n55 = feedback-in #3(w130) -> ()
    n56 = call "Team and Side.vi"("Lado"=w109, "Time"=w110, "field defense"=w102, "Comm RX FPS"=w107, "Game Status"=w130, "Field State Input"=w113) -> ("IA State"=w127:T31)  [unwired: 5 in]
    n57 = call "EventGenerator.vi"("D bola anda"="D bola anda", "Dist Para Toque"="D toque", "Tol para ang posse"="Tol ang posse", "Dist Para posse"="D posse", "IA State Input"=w127, "lado, readius, stretch"=w102) -> ("IA State Output"=w126:T31)  [unwired: 5 in]
    n58 = call <extravilib>:"Write.vi"("element"=w102) -> ("channel"=w103:T42)  [unwired: 8 in, 2 out]
    n59 = call <extravilib>:"Write.vi"("element"=w102) -> ("channel"=w122:T42)  [unwired: 8 in, 2 out]
    n60 = call "Ref Est.vi"("IA State Input"=w126) -> ("IA command"=→"IA command":T9, "IA State Output"=w121:T31)  [unwired: 9 in]
    n61 = call <extravilib>:"Write.vi"("element"=w102) -> ("channel"=w101:T42)  [unwired: 8 in, 2 out]
    n62 = call <extravilib>:"Read.vi"("channel"=w105) -> ("element"=w104:bool[])  [unwired: 5 in, 5 out]
    n63 = call "EventPassState.vi"("TestPasse"=w104, "IA State Input"=w121) -> ("Direct\nkick"=→"Direct\nkick":bool, "IA State Output"=w118:T31, "Pass State"=→"Pass":bool)  [unwired: 6 in, 1 out]
    n64 = call "FuturePose.vi"("IA State Input"=w118) -> ("output cluster"=w119:T31)  [unwired: 10 in]
    n65 = call <extravilib>:"Write.vi"("element"=w119) -> ("channel"=w129:T43)  [unwired: 8 in, 2 out]
  }
  n66 = while {
    shift-right: [w150] -> _
    shift-left: 0.5 ("New Scale") -> [w146]
    shift-right: [w149] -> _
    shift-left: TRUE ("AutoScale Out") -> [w148]
    tunnel: w4 -> [w145]
    tunnel: w5 -> [w143]
    stop <- FALSE stop-if-true
    # "Wait necessario\npara 25 FPS"
    # "Draw Field"
    n67 = event shown="[0] \"2D Picture\": Mouse Wheel" {
      selector: _ -> [_ _]
      dyn-events: _ -> [_ _]
      timeout: 0 -> [_ _]
      tunnel: [w152 1.0] -> w139
      event "2D Picture": Mouse Wheel {
        n68 = event-data() -> ("Delta"=w156:i32)  [unwired: 1 in]
        n69 = Greater Than 0?(x=w156) -> (x > 0?=w155:bool)
        n70 = Select(t=1.2, s=w155, f=0.8) -> (s? t:f=w152:dbl)
      }
      event Timeout {
        n71 = event-data() -> ()  [unwired: 1 in, 3 out]
      }
    }
    n72 = global read "PreviousState.vi" "IA State Output"() -> (w142:T31)
    n73 = call "Field.vi"("channel 2"=w145, "Draw Targets?"="Draw Targets?", "AutoScale"=w148, "IA State Output"=w142, "Zoom"=w139, "Scale mm/pixel"=w146, "channel"=w143) -> ("Scale Out"=w150:dbl, "2D Picture"=→"2D Picture":picture, "AutoScale Out"=w149:bool)  [unwired: 2 in]
    n74 = Wait (ms)(milliseconds to wait=u32 40) -> ()  [unwired: 1 out]
  }
  n75 = while {
    tunnel: w17 -> [w163]
    tunnel: [w162] -> w16
    tunnel: w12 -> [w160]
    stop <- FALSE stop-if-true
    # "Role Decision"
    n76 = call <extravilib>:"Read.vi"("channel"=w160) -> ("element"=w159:bool)  [unwired: 5 in, 5 out]
    n77 = call "Role Decisors Selector.vi"("Pinned"="Pinned", "Modo Teste ?"=w159, "Qtd Min p/ Stk"="Qtd Min p/ Stk", "Role Decisor"="Role Decisor", "channel"=w163) -> ("channel"=w162:T43)  [unwired: 5 in, 1 out]
  }
  n78 = while {
    tunnel: w16 -> [w189]
    tunnel: [w188] -> w20
    tunnel: w15 -> [w185]
    tunnel: [w176] -> w9
    tunnel: [w172] -> w12
    tunnel: [w170] -> w11
    stop <- FALSE stop-if-true
    # "Role Playing"
    n79 = Unbundle By Name("test module") -> ("Modo Teste?"=w174:bool)
    n80 = call "FPS Counter.vi"() -> ("Numeric"=→"Role Playing \nFPS":dbl)  [unwired: 11 in]
    n81 = feedback #4() -> (w173:bool)  [unwired: 1 in]
    n82 = call <extravilib>:"Write.vi"("element"=w173) -> ("channel"=w172:T44)  [unwired: 8 in, 2 out]
    n83 = feedback-in #4(w174) -> ()
    n84 = call "FPS Counter.vi"() -> ("Numeric"=→"Intel FPS":dbl)  [unwired: 11 in]
    n85 = call "Role Playing Simple.vi"(0:"channel"=w189, "AI Parameters"="AI Parameters", "Mais perigoso/segundo mais perigoso"="Mais perigoso/segundo\nmais perigoso", 5:"channel"=w185, "GoTo Navigation"="GoTo Navigation", "test module"="test module", "Debug"="Debug", "atacando ao contrário?"="atacando ao contrário?", "Defesa nova/antiga"="Defesa nova/antiga") -> ("channel"=w188:T43, "IA State Output"=w168:T31, "ball"=→"ball":dbl, "Robot"=→"bot velocity":dbl)  [unwired: 2 in, 1 out]
    n86 = feedback #5() -> (w179:T31)  [unwired: 1 in]
    n87 = global write "PreviousState.vi" "IA State Output"(w179) -> ()
    n88 = feedback-in #5(w168) -> ()
    n89 = call "IA To GUI Robot.vi"("Output IA"=w168) -> ("GUI Robot Array"=→"GUI Robot Array":T11[])  [unwired: 10 in]
    n90 = call <extravilib>:"Write.vi"("element"="atacando ao contrário?") -> ("channel"=w176:T44)  [unwired: 8 in, 2 out]
    n91 = call <extravilib>:"Write.vi"("element"=w168) -> ("channel"=w170:T43)  [unwired: 8 in, 2 out]
    n92 = call "GeradorDegrau.vi"("IA State Input"=w168, "Robô"="Robô", "Liga/Desliga"="Liga/Desliga") -> ()  [unwired: 9 in]
  }
  n93 = while {
    tunnel: [w215] -> w8
    tunnel: [w214] -> w7
    tunnel: w6 -> [w213]
    tunnel: [w198] -> w10
    tunnel: w11 -> [w195]
    tunnel: w9 -> [w193]
    stop <- FALSE stop-if-true
    # "grSim Replacement"
    n94 = call <extravilib>:"Read.vi"("channel"=w195) -> ("element"=w210:T31)  [unwired: 5 in, 5 out]
    n95 = call <extravilib>:"Read.vi"("channel"=w213) -> ("element"=w209:i32[])  [unwired: 5 in, 5 out]
    n96 = call <extravilib>:"Read.vi"("channel"=w193) -> ("element"=w194:bool)  [unwired: 5 in, 5 out]
    n97 = case shown="True" "Test Mode On" {
      tunnel: [cluster{"robots":T14[], "ball":T15} {"robots"=[], "ball"={"x"=0.0, "y"=0.0, "vx"=0.0, "vy"=0.0}} ("grSim replacement") w234] -> w211
      tunnel: w210 -> [_ w233]
      tunnel: w209 -> [_ w232]
      tunnel: "id" -> [_ w231]
      tunnel: "Generate new random points" -> [_ w230]
      tunnel: "Test Mode On" -> [_ w229]
      tunnel: "Number of Points" -> [_ w228]
      tunnel: "reset" -> [_ w227]
      tunnel: "Replace Robots" -> [_ w226]
      tunnel: [_ w225] -> w203
      tunnel: [FALSE ("Completed Generation") w224] -> w202
      tunnel: "Test Attacker" -> [_ w223]
      tunnel: "Modulo Velocidade" -> [_ w222]
      tunnel: [FALSE ("Replace active") w221] -> w191
      tunnel: "Test Passe" -> [_ w220]
      tunnel: w194 -> [_ w219]
      frame False {
      }
      frame True {
        n98 = call "grSim_ReplacementTester.vi"("Generate new random points"=w230, "IA State"=w233, "Atacando contra?"=w219, "Test Attacker"=w223, "id"=w231, "Field defense"=w232, "Test Mode On"=w229, "Number of Points"=w228, "Modulo Velocidade"=w222, "Test Passe"=w220, "reset"=w227, "Replace Robots"=w226) -> ("grSim replacement"=w234:cluster{"robots":T14[], "ball":T15}, "Replace active"=w221:bool, "kick num"=w225:i32, "Completed Generation"=w224:bool)  [unwired: 4 in]
      }
    }
    "Completed Generation" <- w202
    "kick num" <- w203
    n99 = Build Array("Test Passe", w191) -> (w197:bool[])
    n100 = feedback-in #6(w197) -> ()
    n101 = feedback #6() -> (w196:bool[])  [unwired: 1 in]
    n102 = call <extravilib>:"Write.vi"("element"=w196) -> ("channel"=w198:T45)  [unwired: 8 in, 2 out]
    n103 = call <extravilib>:"Write.vi"("element"=w191) -> ("channel"=w215:T44)  [unwired: 8 in, 2 out]
    n104 = call <extravilib>:"Write.vi"("element"=w211) -> ("channel"=w214:T46)  [unwired: 8 in, 2 out]
  }
  n105 = while {
    tunnel: w20 -> [w252]
    tunnel: w8 -> [w239]
    tunnel: w7 -> [w236]
    stop <- FALSE stop-if-true
    # "Communication"
    n106 = call <extravilib>:"Read.vi"("channel"=w236) -> ("element"=w237:cluster{"robots":T14[], "ball":T15})  [unwired: 5 in, 5 out]
    n107 = call <extravilib>:"Read.vi"("channel"=w252) -> ("element"=w240:T31)  [unwired: 5 in, 5 out]
    n108 = call <extravilib>:"Read.vi"("channel"=w239) -> ("element"=w238:bool)  [unwired: 5 in, 5 out]
    n109 = call "FPS Counter.vi"() -> ("Numeric"=→"Comm TX FPS":dbl)  [unwired: 11 in]
    n110 = Unbundle By Name(w240) -> ("Received Timestamp"=w248:timestamp, "our_robots"=w235:T32[], "IA Judge.Time"=w251:enum16{"Azul", "Amarelo"})
    n111 = Get Date/Time In Seconds() -> (seconds since 1Jan1904=w247:timestamp)
    n112 = Subtract(x=w247, y=w248) -> (x-y=→"Total Delay":dbl)
    n113 = call "Convert AI Robot to Robot Command.vi"("Input Array"=w235) -> ("Output Array"=w245:T47[])
    n114 = Equal?(x=w251, y=enum16{"Azul", "Amarelo"}."Amarelo") -> (x = y?=w249:bool)
    n115 = case shown="True" "UDP SOS TX" {
      tunnel: w240 -> [_ w257]
      frame False {
      }
      frame True {
        n116 = call "MessageAI_State.vi"("Port: 2"="SOS Port: 2", "Port:"="SOS Port:", "SSL Vision Address:"="SOS Address:", "IA state"=w257) -> ()  [unwired: 8 in]
      }
    }
    n117 = case shown="True" "UDP GrSim TX" {
      tunnel: w249 -> [_ w268]
      tunnel: w245 -> [_ w266]
      tunnel: w238 -> [_ w264]
      tunnel: w237 -> [_ w263]
      frame False {
      }
      frame True {
        n118 = call "grSim Packet Command UDP Test.vi"("grSim replacement"=w263, "replace ball"=w264, "Port:"="Port:", "SSL Vision Address:"="Address:", "isteamyellow"=w268, "Robots"=w266) -> ()  [unwired: 6 in]
        "replace active" <- w264
        "grSim replacement" <- w263
      }
    }
    n119 = case shown="True" "Serial TX" {
      tunnel: w245 -> [_ w258]
      frame False {
      }
      frame True {
        n120 = for {
          tunnel: w258 -> [w262] mode=indexing
          n121 = call "Serial Transmitter.vi"("Porta:"="Porta:", "Robots"=w262) -> ("error out"=→"error out 5":errorcluster)  [unwired: 9 in]
          n122 = Wait (ms)(milliseconds to wait=u32 2) -> ()  [unwired: 1 out]
        }
      }
    }
  }
